vi "Access Launcher.vi"(8 "error in (no error)":errorcluster, 9 "ID":string, 10 "Nested Actor":refnum<class "Actor.lvclass">, 11 "gController in":refnum<class "gController.lvclass">) -> (0 "error out":errorcluster, 2 "Launch Successful?":bool, 3 "gController out":refnum<class "gController.lvclass">)   [LabVIEW 2018, in "Controller.lvlib" / "gController.lvclass"]
uses:
  gController.lvclass
  C:/Program Files (x86)/National Instruments/LabVIEW 2018/vi.lib/MSR Consulting, LLC/General Reuse/SuperActor/SuperActor.lvclass
  <vilib>/ActorFramework/Actor/Actor.lvclass
  <vilib>/MSR Consulting, LLC/General Reuse/SuperActor/SuperActor.lvclass
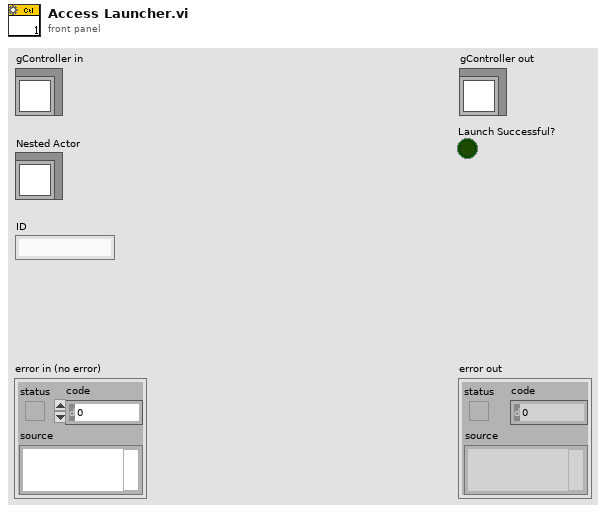
[diagram p1: front panel]
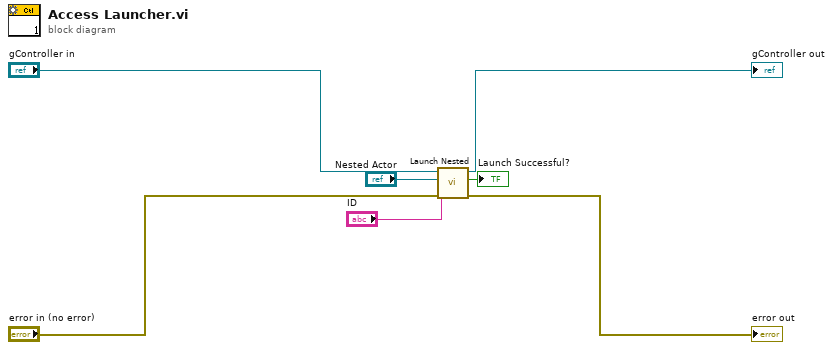
[diagram p0: block diagram]
diagram:
  n1 = call <vilib>:"Launch Nested.vi"("error in"="error in (no error)", "ID"="ID", "Nested Actor"="Nested Actor", "SuperActor in"="gController in") -> ("error out"=→"error out":errorcluster, "Launch Successful?"=→"Launch Successful?":bool, "SuperActor out"=→"gController out":refnum<class "gController.lvclass">)  [unwired: 5 in]
